vi "CField.vi"(0 "VisaCluster":T1, 7 "CField":bool, 11 "error in (no error)":errorcluster) -> (4 "VisaCluster":T1, 6 "Answer":string, 8 "CField 2":bool, 15 "error out":errorcluster)   [LabVIEW 2014, in "FH 55.lvlib"]
doc: "This VI sets the Field Correction ON or OFF.\n\nDurch dises VI wird die Linearitäts-Korrektur an oder ausgeschaltet. Voraussetzung ist, dass im Sonden-Eeprom Korrekturdaten vorliegen. Die Wahl \"OFF\" führt dazu, dass diese Tabelle ignoriert wird. Die Korrekturdaten sind automatisch eingeschaltet."
uses:
  FH 55.lvlib
  TypeDef/VisaCluster.ctl
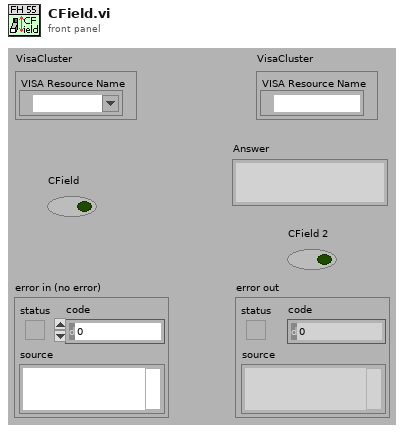
[diagram p1: front panel]
types:
  T1 = typedef "FH 55.lvlib/VisaCluster.ctl" = cluster{"VISA Resource Name":refnum<visa-resource-name>}
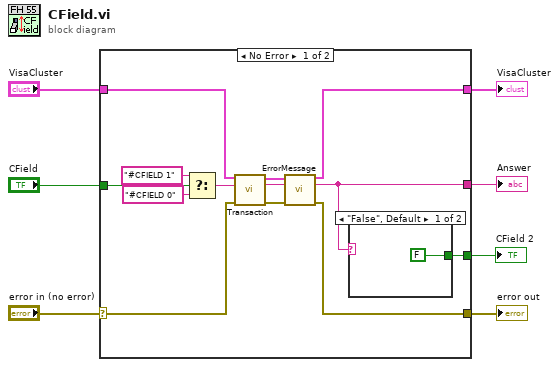
[diagram p0: block diagram]
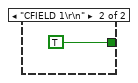
[diagram p2: hidden frame]
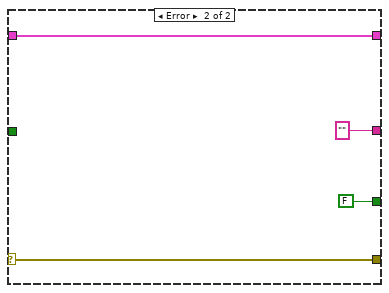
[diagram p3: hidden frame]
diagram:
  n1 = case shown="No Error" "error in (no error)" {
    selector: "error in (no error)" -> [w13 w25]
    tunnel: "VisaCluster" -> [w15 w26]
    tunnel: "CField" -> [w20 _]
    tunnel: [w17 w26] -> w3
    tunnel: [w16 w25] -> w5
    tunnel: [w9 ""] -> w4
    tunnel: [w8 FALSE] -> w1
    frame No Error {
      n2 = Select(t="#CFIELD 1", s=w20, f="#CFIELD 0") -> (s? t:f=w14:string)
      n3 = call "Transaction.vi"("VisaCluster"=w15, "Command"=w14, "error in (no error)"=w13) -> ("VisaCluster"=w10:T1, "Answer"=w11:string, "error out"=w12:errorcluster)  [unwired: 9 in, 1 out]
      n4 = call "ErrorMessage.vi"("VisaCluster"=w10, "Message In"=w11, "error in (no error)"=w12) -> ("VisaCluster"=w17:T1, "Message Out"=w9:string, "error out"=w16:errorcluster)  [unwired: 10 in]
      n5 = case shown="\"False\", Default" w9 {
        tunnel: [FALSE TRUE] -> w8
        frame "False", Default {
        }
        frame "CFIELD 1\r\n" {
        }
      }
    }
    frame Error {
    }
  }
  "error out" <- w5
  "Answer" <- w4
  "VisaCluster" <- w3
  "CField 2" <- w1
